vi "Read Variance.vi"(8 "error in (no error)":errorcluster, 11 "Moving_Statistic in":refnum<class "Moving_Statistic.lvclass">) -> (0 "error out":errorcluster, 2 "Variance":dbl, 3 "Moving_Statistic out":refnum<class "Moving_Statistic.lvclass">)   [LabVIEW 2021, in "Moving_Statistic.lvclass"]
uses:
  Moving_Statistic.lvclass
  Moving_Statistic.lvclass/Moving_Statistic.ctl
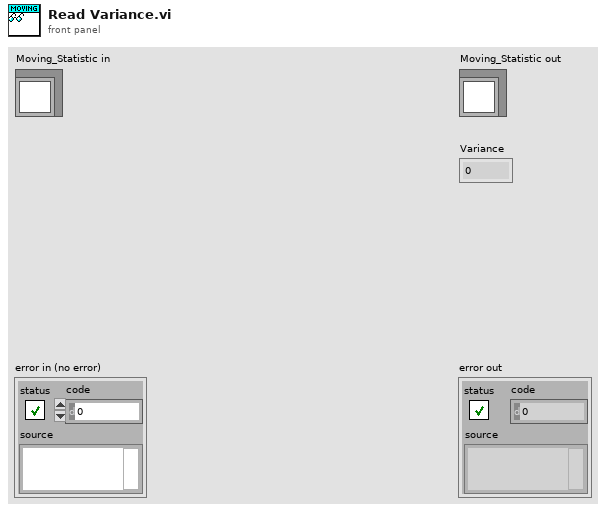
[diagram p1: front panel]
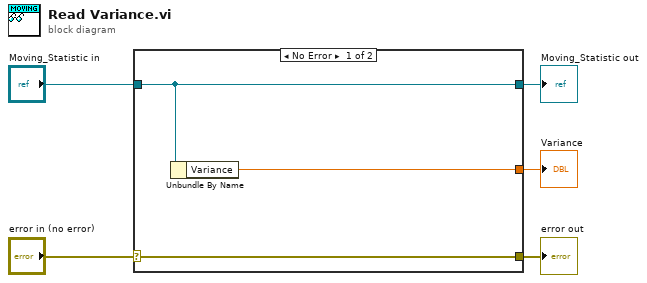
[diagram p0: block diagram]
diagram:
  n1 = case shown="No Error" "error in (no error)" {
    selector: "error in (no error)" -> [w8 w9]
    tunnel: [w8 w9] -> w4
    tunnel: [w7 w10] -> w2
    tunnel: "Moving_Statistic in" -> [w7 w10]
    tunnel: [w6 _] -> w1
    frame No Error {
      n2 = Unbundle By Name(w7) -> ("Variance"=w6:dbl)
    }
    frame Error {
    }
  }
  "error out" <- w4
  "Moving_Statistic out" <- w2
  "Variance" <- w1
